vi "Init Values.vi"(8 "error in (no error)":errorcluster, 11 "Dynamic Combobox in":refnum<class "Dynamic Combobox.lvclass">) -> (0 "error out":errorcluster, 3 "Dynamic Combobox out":refnum<class "Dynamic Combobox.lvclass">)   [LabVIEW 2020, in "Dynamic Combobox.lvlib" / "Dynamic Combobox.lvclass"]
uses:
  Dynamic Combobox.lvclass
  Dynamic Combobox.lvclass/Dynamic Combobox.ctl
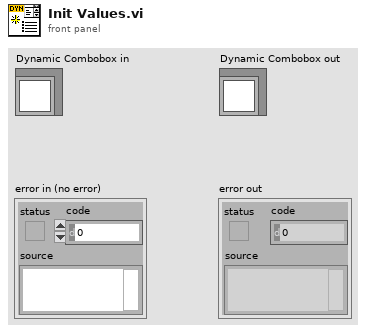
[diagram p1: front panel]
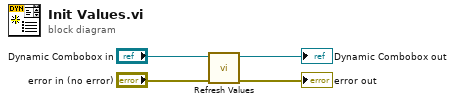
[diagram p0: block diagram]
diagram:
  n1 = call "Refresh Values.vi"("error in (no error)"="error in (no error)", "Dynamic Combobox in"="Dynamic Combobox in") -> ("error out"=→"error out":errorcluster, "Dynamic Combobox out"=→"Dynamic Combobox out":refnum<class "Dynamic Combobox.lvclass">)  [unwired: 8 in]
